vi "Set Defaults.vi"(11 "NewEntityTemplate in":refnum<class "Player.lvclass">) -> (3 "NewEntityTemplate out":refnum<class "Player.lvclass">)   [LabVIEW 2020, in "Test.lvlib" / "Player.lvclass"]
uses:
  Player.lvclass
  Player.lvclass/Player.ctl
  <vilib>/IlluminatedG/IG Conditum Base/Conditum/Columns/String/String.lvclass
  <vilib>/IlluminatedG/IG Conditum Base/Conditum/Columns/Double/Double.lvclass
  <vilib>/IlluminatedG/IG Conditum Base/Conditum/Columns/Boolean/Boolean.lvclass
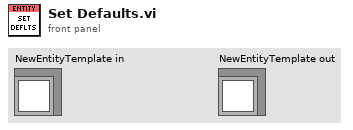
[diagram p1: front panel]
types:
  T1 = typedef "Test.lvlib/Player.lvclass/Columns.ctl" = cluster{"Name":refnum<class "String.lvclass">, "Score":refnum<class "Double.lvclass">, "Active":refnum<class "Boolean.lvclass">}
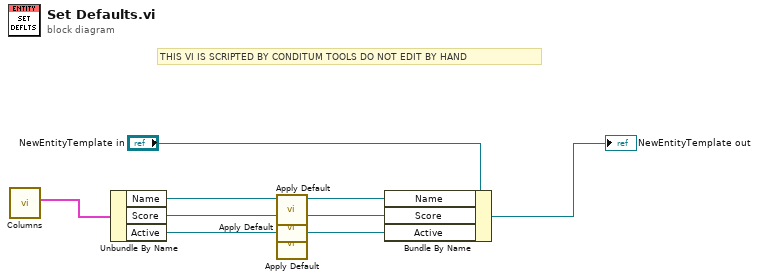
[diagram p0: block diagram]
diagram:
  # "THIS VI IS SCRIPTED BY CONDITUM TOOLS DO NOT EDIT BY HAND"
  n1 = call "Columns.vi"() -> ("Columns"=w9:T1)  [unwired: 11 in]
  n2 = Unbundle By Name(w9) -> ("Name"=w6:refnum<class "String.lvclass">, "Score"=w5:refnum<class "Double.lvclass">, "Active"=w4:refnum<class "Boolean.lvclass">)
  n3 = call-dynamic "Apply Default.vi"("String in"=w6) -> ("String out"=w3:refnum<class "String.lvclass">)  [unwired: 10 in]
  n4 = call-dynamic "Apply Default.vi"("Double in"=w5) -> ("Double out"=w2:refnum<class "Double.lvclass">)  [unwired: 10 in]
  n5 = call-dynamic "Apply Default.vi"("Boolean in"=w4) -> ("Boolean out"=w1:refnum<class "Boolean.lvclass">)  [unwired: 10 in]
  n6 = Bundle By Name(cluster="NewEntityTemplate in", "Name"=w3, "Score"=w2, "Active"=w1) -> (→"NewEntityTemplate out":refnum<class "Player.lvclass">)
